vi "RunAnalogRead.vi"() -> ()   [LabVIEW 2014]
uses:
  daq_channel_read_parameter.ctl
  <vilib>/Platform/TimedLoop/XDataNode/timing_clust.ctl
  <vilib>/Platform/TimedLoop/XDataNode/nitl_modes.ctl
  <vilib>/Platform/TimedLoop/XDataNode/wakeup.ctl
  <vilib>/platform/TimedLoop/XDataNode/XDataNode.xnode
  <vilib>/Platform/TimedLoop/XDataNode/XDNodeRunTimeDep.lvlib
panel:
  out "Numeric":i32
  in  "data2plot":dbl[](array[numeric])
  in  "channelSamFreq_Hz":dbl
  in  "displayTime_Sec":dbl
  out "signal":waveform(dbl)(graph)
  in  "chanellParaCluster":T1={"audioOffState_V"=0.0, "audioFilterPeriod_uS"=50000, "audioThreshold_V"=0.0, "vsThreshold_V"=0.0, "vsFilterPeriod_uS"=0, "lickThreshold_V"=0.0} {"vsFilterPeriod_uS" format="%#1.6f"; "audioFilterPeriod_uS" format="%#1.6f"}
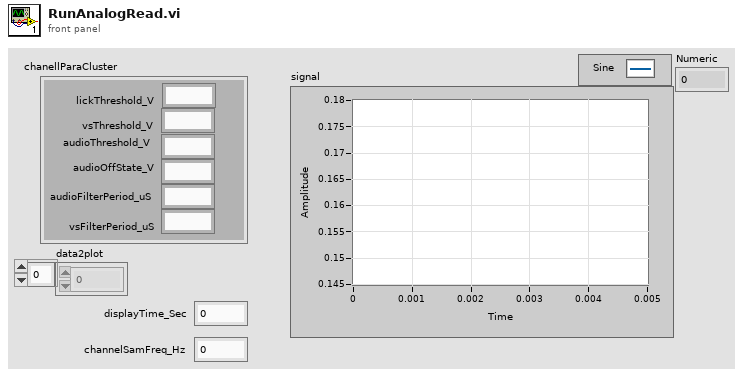
[diagram p1: front panel]
types:
  T1 = typedef "daq_channel_read_parameter.ctl" = cluster{"audioOffState_V":fxp<+/-,16,5>, "audioFilterPeriod_uS":i32, "audioThreshold_V":fxp<+/-,16,5>, "vsThreshold_V":fxp<+/-,16,5>, "vsFilterPeriod_uS":i32, "lickThreshold_V":fxp<+/-,16,5>}
  T2 = typedef "XDNodeRunTimeDep.lvlib/timing_clust.ctl" = cluster{"Expected End [f-1]":u64, "Actual End [f-1]":u64, "Finished Late? [f-1]":bool, "Expected End [i-1]":u64, "Actual End [i-1]":u64, "Finished Late? [i-1]":bool, "Expected Start [i]":u64, "Actual Start [i]":u64, "Expected Start [f]":u64, "Actual Start [f]":u64, "Source Name":string, "Structure Name":string, "Period":i64, "Deadline":i64, "Offset":i64, "Start":i64, "Priority":i32, "Timeout":i32, "Mode":T3, "Wakeup Reason":T4, "Error":errorcluster, "Source Type":string, "Secondary Source Type":string, "Global End Time":u64, "Global Start Time":u64, "Frame Duration":u64, "Iteration Duration":u64, "Assigned CPU":i32, "I/O Scan Engine Mode":u32}
  T3 = typedef "XDNodeRunTimeDep.lvlib/nitl_modes.ctl" = enum32{"No Change", "Process missed periods, maintain original phase", "Discard missed periods, maintain original phase", "Process missed periods, ignore original phase", "Discard missed periods, ignore original phase"}
  T4 = typedef "XDNodeRunTimeDep.lvlib/wakeup.ctl" = enum32{"Normal", "Aborted", "Asynchronous wakeup", "Timing source error", "Timed loop error", "Timeout"}
  T5 = cluster{"leftLick":dbl, "rightLick":dbl, "visualStimuli2":dbl, "tone":dbl, "visualStimuli1":dbl}
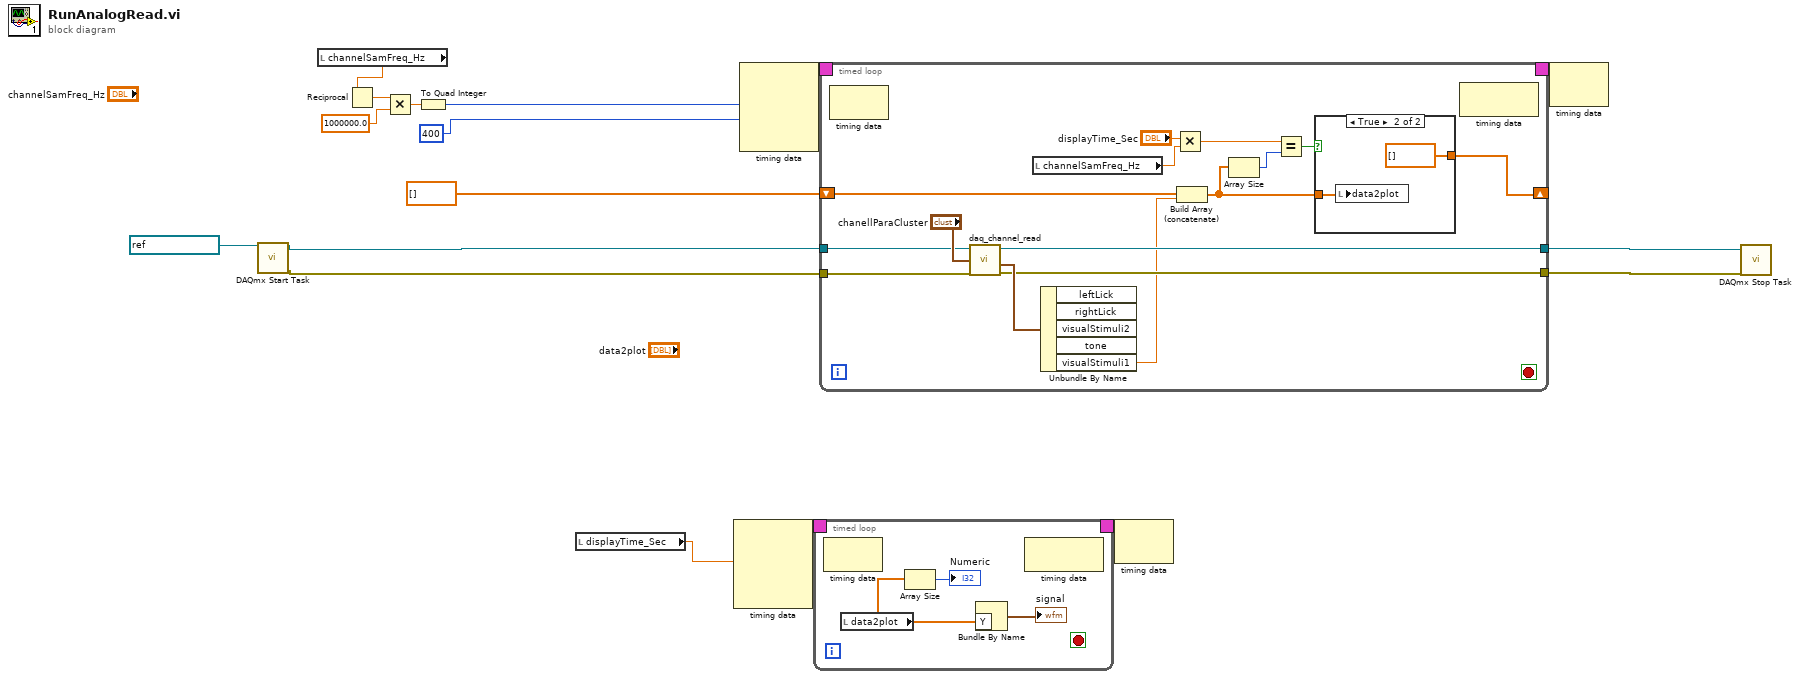
[diagram p0: block diagram]
diagram:
  n1 = call <vilib>:"DAQmx Start Task.vi"("task/channels in"=refnum<k21> "analogRead" ("DAQmx Task Name")) -> ("task out"=w16:refnum<k21>, "error out"=w15:errorcluster)  [unwired: 13 in]
  n2 = local read "channelSamFreq_Hz"() -> (w9:dbl)
  n3 = Reciprocal(x=w9) -> (1/x=w8:dbl)
  n4 = Multiply(x=w8, y=1000000.0) -> (x*y=w6:dbl)
  n5 = To Quad Integer(1:w6) -> (0:w5:i64)
  n6 = local read "displayTime_Sec"() -> (w1:dbl)
  n7 = node-c288(w1) -> (w4:T2)  [unwired: 3 in]
  n8 = node-c288(w5, 400) -> (w12:T2)  [unwired: 2 in]
  n9 = timed-loop {
    timing: w4 -> [_]
    timing-out: [_] -> w3
    stop <- _ stop-if-true
    n10 = node-c288() -> ()  [unwired: 1 in, 1 out]
    n11 = local read "data2plot"() -> (w19:dbl[])
    n12 = Array Size(array=w19) -> (size(s)=→"Numeric":i32)
    n13 = Bundle By Name("Y"=w19) -> (→"signal":waveform(dbl))  [unwired: 1 in]
    n14 = node-c288() -> ()  [unwired: 1 in, 1 out]
  }
  n15 = timed-loop {
    timing: w12 -> [_]
    timing-out: [_] -> w11
    tunnel: w16 -> [w36]
    tunnel: w15 -> [w35]
    tunnel: [w34] -> w14
    tunnel: [w32] -> w13
    shift-right: [w25] -> _
    shift-left: dbl[] [] ("array type (2D Dbl)") -> [w31]
    stop <- _ stop-if-true
    n16 = node-c288() -> ()  [unwired: 1 in, 1 out]
    n17 = call "daq_channel_read.vi"("DAQmxTaskIn"=w36, "chanellParaCluster"="chanellParaCluster", "error in (no error)"=w35) -> ("DAQmxTaskOut"=w34:refnum<k21>, "channelOutCluster_rawData"=w33:T5, "error out"=w32:errorcluster)  [unwired: 1 out]
    n18 = local read "channelSamFreq_Hz"() -> (w29:dbl)
    n19 = Unbundle By Name(w33) -> ("visualStimuli1"=w24:dbl)  [unwired: 4 out]
    n20 = Multiply(x="displayTime_Sec", y=w29) -> (x*y=w28:dbl)
    n21 = Build Array (concatenate)(w31, w24) -> (w23:dbl[])
    n22 = Array Size(array=w23) -> (size(s)=w27:i32)
    n23 = Equal?(x=w28, y=w27) -> (x = y?=w26:bool)
    n24 = case shown="True" w26 {
      tunnel: [w38 dbl[] [] ("array type (2D Dbl)")] -> w25
      tunnel: w23 -> [w38 w39]
      frame False {
      }
      frame True {
        n25 = local write "data2plot"(w39) -> ()
      }
    }
    n26 = node-c288() -> ()  [unwired: 1 in, 1 out]
  }
  n27 = node-c288(w3) -> ()  [unwired: 1 out]
  n28 = node-c288(w11) -> ()  [unwired: 1 out]
  n29 = call <vilib>:"DAQmx Stop Task.vi"("task/channels in"=w14, "error in"=w13) -> ()  [unwired: 12 in, 2 out]
